vi "callback.vi"(4 "callback settings":T1, 6 "CtlRef":refnum<vi>, 7 "Event Common Data":cluster{"Source":T2, "Type":T3, "Time":u32} {"Source" items=["LabVIEW UI"=0, "ActiveX"=1, "User Event"=25]}) -> ()   [LabVIEW 2013, in "displayable.lvclass"]
uses:
  displayable.lvclass
  <vilib>/event_ctls.llb/eventsource.ctl
  <vilib>/event_ctls.llb/lveventtype.ctl
  callback settings.ctl
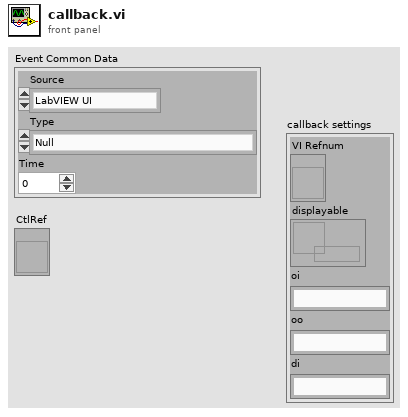
[diagram p1: front panel]
types:
  T1 = typedef "displayable.lvclass/callback settings.ctl" = cluster{"VI Refnum":refnum<vi>, "displayable":refnum<data-value>, "oi":string, "oo":string, "di":string}
  T2 = typedef "eventsource.ctl" = u32
  T3 = typedef "lveventtype.ctl" = enum32{"Null", "Timeout", "Annotation Menu Selection", "Annotation Menu Selection?", "App Instance Close", "App Instance Close?", "Autoscale Range Change", "Bookmark Info Change", "Cell Edit", "Cell Edit?", "Cursor Grab", "Cursor Grab?", "Cursor Menu Selection", "Cursor Menu Selection?", "Cursor Move", "Cursor Release", "Data Change", "Direction Change", "Display State Change", "Drag Ended", "Drag Enter", "Drag Leave", "Drag Over", "Drag Source Update", "Drag Starting", "Drag Starting?", "Drop", "Exec State Change", "Key Down", "Key Down?", "Key Repeat", "Key Repeat?", "Key Up", "Listbox Double Click", "Menu Activation?", "Menu Selection (App)", "Menu Selection? (App)", "Menu Selection (User)", "Mouse Down", "Mouse Down?", "Mouse Enter", "Mouse Leave", "Mouse Move", "Mouse Up", "Mouse Wheel", "NI Security User Change (App)", "Pane Size", "Panel Close", "Panel Close?", "Panel Resize", "Plot Attribute Change", "Scale Range Change", "Shortcut Menu Activation?", "Shortcut Menu Selection (App)", "Shortcut Menu Selection? (App)", "Shortcut Menu Selection (User)", "Tree Double Click", "Tree Drag", "Tree Drag?", "Tree Drop", "Tree Drop?", "Tree Item Close", "Tree Item Close?", "Tree Item Open", "Tree Item Open?", "User Event", "Value Change"}
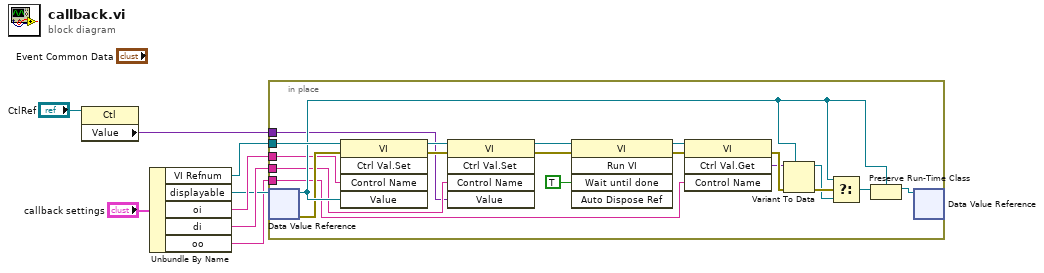
[diagram p0: block diagram]
diagram:
  n1 = property class="Ctl"(reference="CtlRef") -> ("Value"=w5:variant)  [unwired: 1 in, 2 out]
  n2 = Unbundle By Name("callback settings") -> ("VI Refnum"=w6:refnum<vi>, "displayable"=w2:refnum<data-value>, "oi"=w3:string, "di"=w4:string, "oo"=w1:string)
  n3 = in-place {
    in-place-border: w6 -> [w27]
    in-place-border: w5 -> [w9]
    in-place-border: w4 -> [w10]
    in-place-border: w3 -> [w17]
    in-place-border: w1 -> [w11]
    n4 = in-place-dvr #1(w2) -> (w23:refnum<class "displayable.lvclass">, w18:errorcluster)
    n5 = invoke class="VI" method="Ctrl Val.Set"(reference=w27, error in=w18, "Control Name"=w17, "Value"=w23) -> (reference out=w22:refnum<vi>, error out=w19:errorcluster)  [unwired: 1 in, 3 out]
    n6 = invoke class="VI" method="Ctrl Val.Set"(reference=w22, error in=w19, "Control Name"=w10, "Value"=w9) -> (reference out=w21:refnum<vi>, error out=w20:errorcluster)  [unwired: 1 in, 3 out]
    n7 = invoke class="VI" method="Run VI"(reference=w21, error in=w20, "Wait until done"=TRUE ("Wait Until Done")) -> (reference out=w15:refnum<vi>, error out=w14:errorcluster)  [unwired: 2 in, 3 out]
    n8 = invoke class="VI" method="Ctrl Val.Get"(reference=w15, error in=w14, "Control Name"=w11) -> (error out=w13:errorcluster, "Get Control Value Variant"=w12:variant)  [unwired: 1 in, 2 out]
    n9 = Variant To Data(error in=w13, type=w23, Variant=w12) -> (data=w16:refnum<class "displayable.lvclass">, error out=w25:errorcluster)
    n10 = Select(t=w23, s=w25, f=w16) -> (s? t:f=w26:refnum<class "displayable.lvclass">)
    n11 = Preserve Run-Time Class(object in=w26, 2:w23) -> (object out=w24:refnum<class "displayable.lvclass">)  [unwired: 1 in, 1 out]
    n12 = in-place-dvr #1(w24) -> ()  [unwired: 2 out]
  }
